vi "SGSA_Sweep_record_ALL.vi"() -> ()   [LabVIEW 2023, in "SG_SA.lvlib"]
uses:
  SG_SA.lvlib
  Clover_Cell.lvlib
panel:
  in  "Air_Loss":dbl=8.0
  in  "Cable_Loss":dbl=8.0
  in  "WaitingTime(ms)":u32=1000
  in  "FileNote":string
  in  "TRXmode":u16(ring)=1 items=["QUERY_TELEM_2 (V)"=2, "QUERY_TELEM_1 (H)"=1]
  out "SG Power (dBm)":i32
  in  "Stop Power":i32=8
  in  "Start Power":i32=-40
  in  "SG":refnum<visa-resource-name>="TCPIP0::192.168.100.200::inst0::INSTR"
  in  "SA":refnum<visa-resource-name>="TCPIP0::192.168.100.230::inst0::INSTR"
  in  "AvgTimes":i32=5
  out "Spectrum Data":dbl[](graph)
  out "AiP_8":dbl format="%#2.2f"
  out "AiP_7":dbl format="%#2.2f"
  out "AiP_6":dbl format="%#2.2f"
  out "AiP_5":dbl format="%#2.2f"
  out "AiP_4":dbl format="%#2.2f"
  out "AiP_3":dbl format="%#2.2f"
  out "AiP_2":dbl format="%#2.2f"
  out "AiP_1":dbl format="%#2.2f"
  # "Temperature"
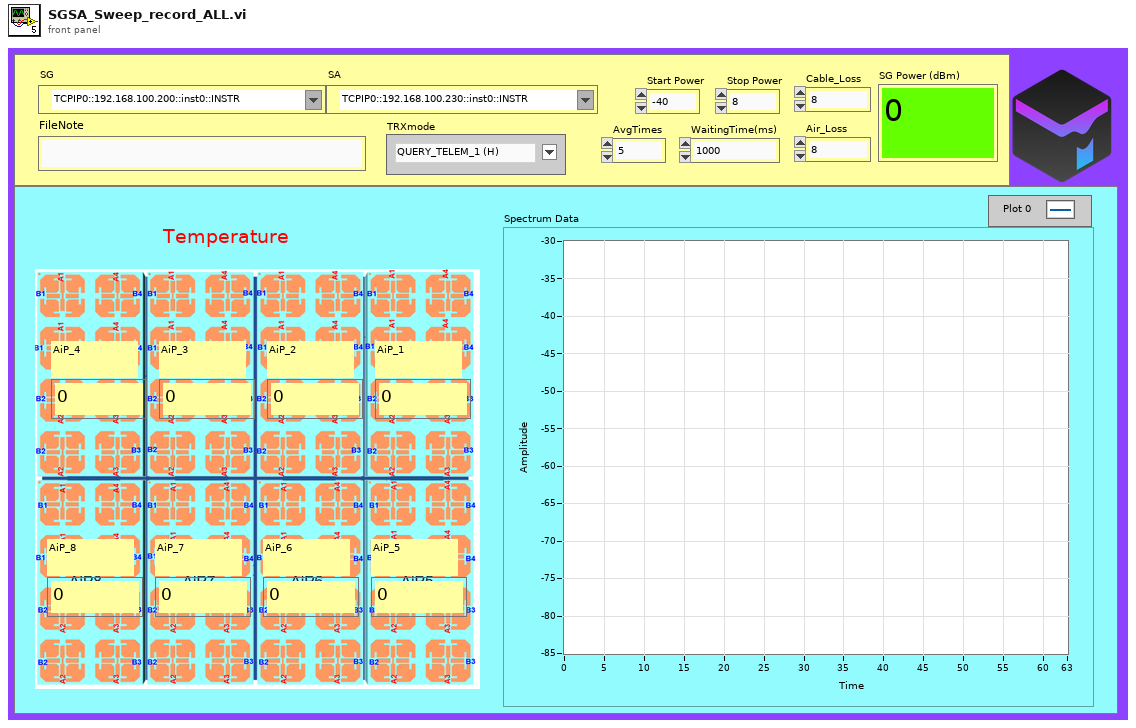
[diagram p1: front panel]
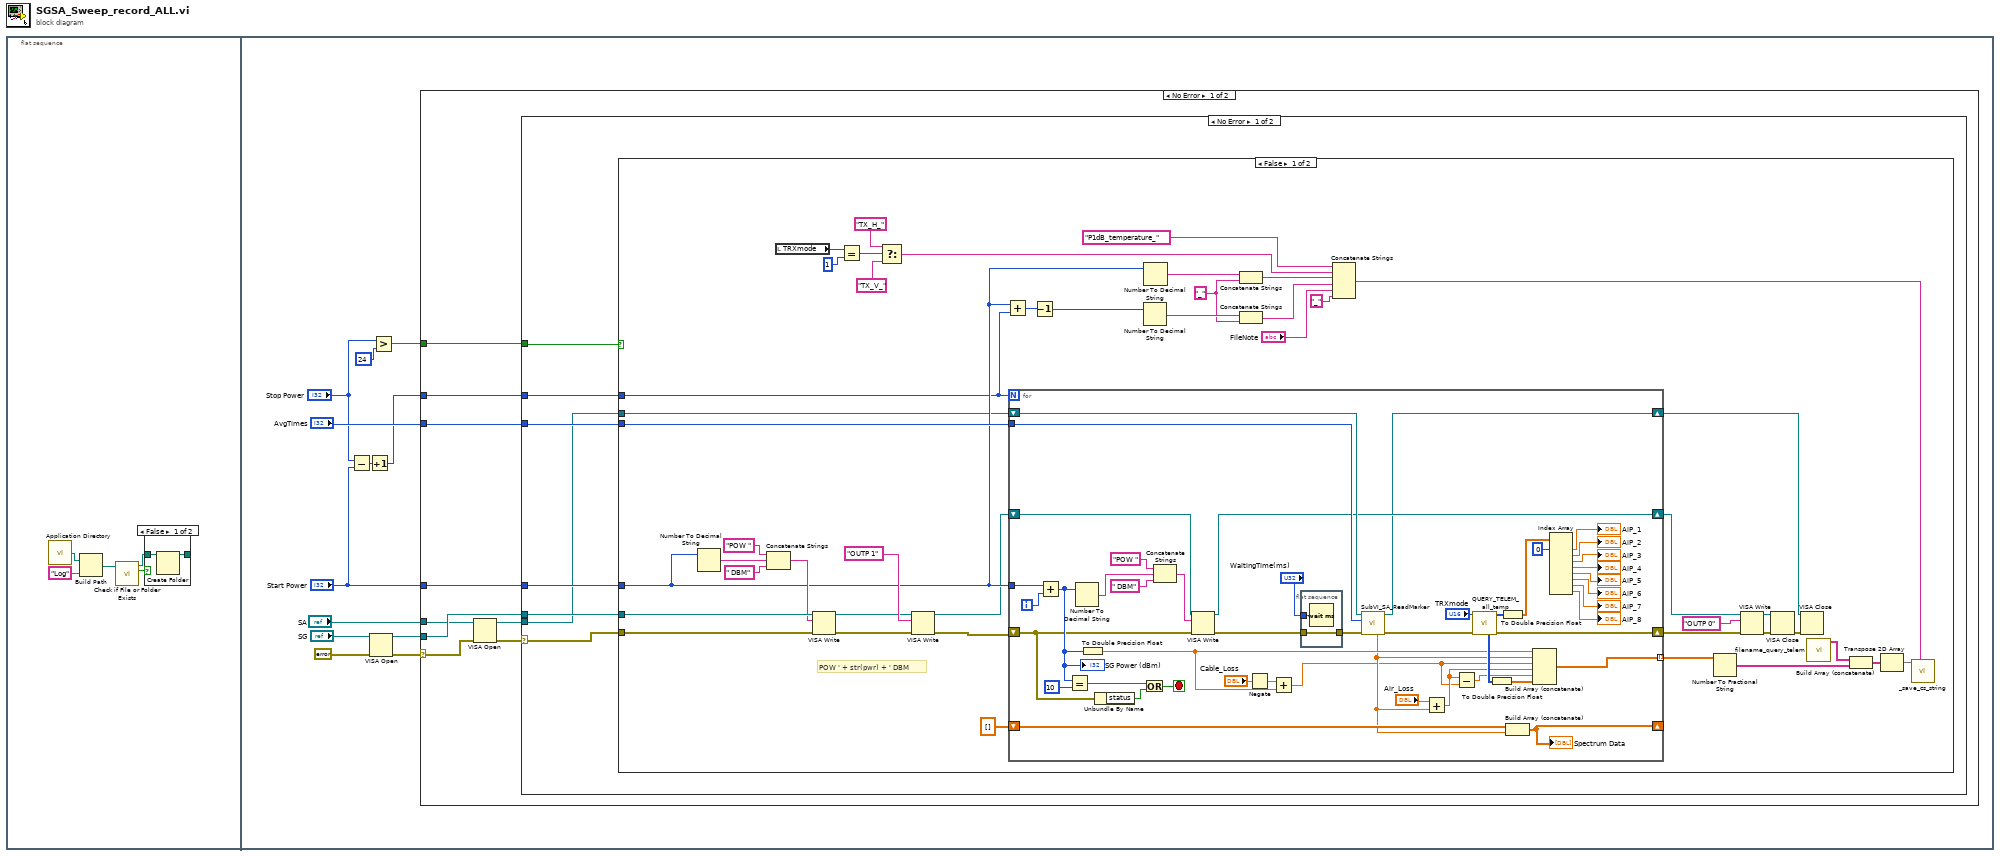
[diagram p0: block diagram]
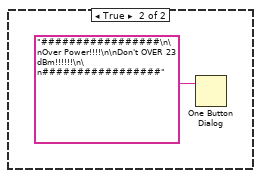
[diagram p3: hidden frame]
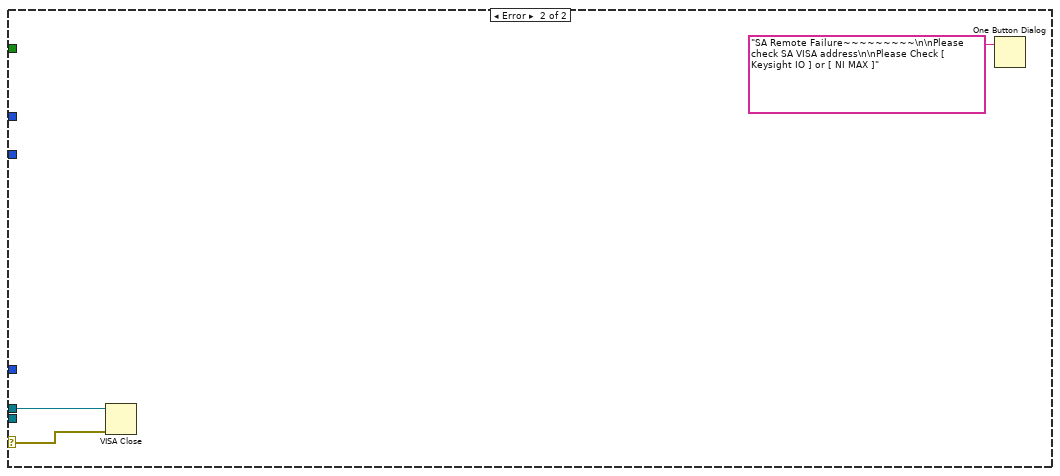
[diagram p4: hidden frame]
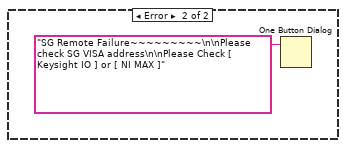
[diagram p5: hidden frame]
diagram:
  n1 = flat-sequence {
    frame #0 {
      n2 = call <vilib>:"Application Directory.vi"() -> ("Application Directory"=w4:path)
      n3 = Build Path(base path=w4, name or relative path="Log") -> (appended path=w1:path)
      n4 = call <vilib>:"Check if File or Folder Exists.vi"("path"=w1) -> ("file or folder exists?"=w3:bool, "dup path"=w2:path)  [unwired: 8 in, 1 out]
      n5 = case shown="False" w3 {
        tunnel: w2 -> [w7 w8]
        tunnel: [w6 w8] -> _
        frame False {
          n6 = Create Folder(path (use dialog)=w7) -> (created path=w6:path)  [unwired: 2 in, 2 out]
        }
        frame True {
        }
      }
    }
    frame #1 {
      n7 = Subtract(x="Stop Power", y="Start Power") -> (x-y=w17:i32)
      n8 = Increment(x=w17) -> (x+1=w16:i32)
      n9 = VISA Open(error in (no error)=errorcluster {"status"=FALSE, "code"=0, "source"=""}, VISA resource name="SG") -> (VISA resource name=w11:refnum<visa-resource-name>, error out=w9:errorcluster)  [unwired: 3 in]
      n10 = Greater?(x="Stop Power", y=24) -> (0:w20:bool)
      n11 = case shown="No Error" w9 {
        selector: w9 -> [w22 _]
        tunnel: w20 -> [w29 _]
        tunnel: "Start Power" -> [w28 _]
        tunnel: "AvgTimes" -> [w27 _]
        tunnel: w16 -> [w26 _]
        tunnel: w11 -> [w25 _]
        tunnel: "SA" -> [w24 _]
        frame No Error {
          n12 = VISA Open(error in (no error)=w22, VISA resource name=w24) -> (VISA resource name=w23:refnum<visa-resource-name>, error out=w21:errorcluster)  [unwired: 3 in]
          n13 = case shown="No Error" w21 {
            selector: w21 -> [w30 w132]
            tunnel: w29 -> [w36 _]
            tunnel: w28 -> [w35 _]
            tunnel: w27 -> [w34 _]
            tunnel: w26 -> [w33 _]
            tunnel: w25 -> [w32 w133]
            tunnel: w23 -> [w31 _]
            frame No Error {
              n14 = case shown="False" w36 {
                tunnel: w34 -> [w81 _]
                tunnel: w35 -> [w71 _]
                tunnel: w30 -> [w75 _]
                tunnel: w32 -> [w74 _]
                tunnel: w33 -> [w70 _]
                tunnel: w31 -> [w45 _]
                frame False {
                  w61 = "_"
                  # "POW ' + str(pwr) + ' DBM"
                  n15 = Number To Decimal String(number=w71) -> (decimal integer string=w77:string)  [unwired: 1 in]
                  n16 = Concatenate Strings("POW ", w77, " DBM") -> (w72:string)
                  n17 = local read "TRXmode"() -> (w44:u16)
                  n18 = VISA Write(VISA resource name=w74, write buffer=w72, error in (no error)=w75) -> (VISA resource name out=w73:refnum<visa-resource-name>, error out=w76:errorcluster)  [unwired: 1 out]
                  n19 = Equal?(x=w44, y=u16 1) -> (x = y?=w42:bool)
                  n20 = Select(t="TX_H_" ("delimiter (\\t)"), s=w42, f="TX_V_" ("delimiter (\\t)")) -> (s? t:f=w39:string)
                  n21 = VISA Write(VISA resource name=w73, write buffer="OUTP 1", error in (no error)=w76) -> (VISA resource name out=w69:refnum<visa-resource-name>, error out=w68:errorcluster)  [unwired: 1 out]
                  n22 = Add(x=w71, y=w70) -> (x+y=w65:i32)
                  n23 = for {
                    N: w70 -> [_]
                    tunnel: w81 -> [w127]
                    tunnel: w71 -> [w125]
                    tunnel: [w120] -> w53 mode=indexing
                    shift-right: [w116] -> w66
                    shift-left: w68 -> [w100]
                    shift-right: [w113] -> w58
                    shift-left: w69 -> [w112]
                    shift-right: [w96] -> w46
                    shift-left: w45 -> [w128]
                    shift-right: [w91] -> _
                    shift-left: dbl[] [] -> [w92]
                    i -> [w126]
                    stop <- w99 stop-if-true
                    n24 = Add(x=w125, y=w126) -> (x+y=w119:i32)
                    "SG Power (dBm)" <- w119
                    n25 = Equal?(x=w119, y=10) -> (x = y?=w98:bool)
                    n26 = Number To Decimal String(number=w119) -> (decimal integer string=w122:string)  [unwired: 1 in]
                    n27 = To Double Precision Float(number=w119) -> (double precision float=w88:dbl)
                    n28 = Unbundle By Name(w100) -> ("status"=w97:bool)
                    n29 = Or(x=w98, y=w97) -> (x .or. y?=w99:bool)
                    n30 = Concatenate Strings("POW ", w122, " DBM") -> (w121:string)
                    n31 = VISA Write(VISA resource name=w112, write buffer=w121, error in (no error)=w100) -> (VISA resource name out=w113:refnum<visa-resource-name>, error out=w95:errorcluster)  [unwired: 1 out]
                    n32 = Negate(x="Cable_Loss") -> (-x=w89:dbl)
                    n33 = Add(x=w89, y=w88) -> (x+y=w83:dbl)
                    n34 = flat-sequence {
                      tunnel: w95 -> [w130]
                      tunnel: [w130] -> w94
                      tunnel: "WaitingTime(ms)" -> [w129]
                      frame #0 {
                        n35 = Wait (ms)(milliseconds to wait=w129) -> ()  [unwired: 1 out]
                      }
                    }
                    n36 = call "SubVI_SA_ReadMarker.vi"("error in (no error)"=w94, "AvgTimes"=w127, "VISA resource name"=w128) -> ("error out"=w117:errorcluster, "VISA resource name out"=w96:refnum<visa-resource-name>, "Marker Power"=w86:dbl)  [unwired: 5 in, 1 out]
                    n37 = Add(x="Air_Loss", y=w86) -> (x+y=w84:dbl)
                    n38 = Subtract(x=w84, y=w83) -> (x-y=w82:dbl)
                    n39 = call "QUERY_TELEM_all_temp.vi"("error in"=w117, "TRXmode"="TRXmode") -> ("error out"=w116:errorcluster, "Temp_8pcs"=w115:i32[], "all_data"=w101:i32[])  [unwired: 7 in]
                    n40 = To Double Precision Float(number=w101) -> (double precision float=w85:dbl[])
                    n41 = To Double Precision Float(number=w115) -> (double precision float=w111:dbl[])
                    n42 = Build Array (concatenate)(w92, w86) -> (w91:dbl[])
                    "Spectrum Data" <- w91
                    n43 = Build Array (concatenate)(w88, w86, w83, w84, w82, w85) -> (w120:dbl[])
                    n44 = Index Array(array=w111, index #1=0 ("index")) -> (element #1=→"AiP_1":dbl, element #2=→"AiP_2":dbl, element #3=→"AiP_3":dbl, element #4=→"AiP_4":dbl, element #5=→"AiP_5":dbl, element #6=→"AiP_6":dbl, element #7=→"AiP_7":dbl, element #8=→"AiP_8":dbl)  [unwired: 7 in]
                  }
                  n45 = Decrement(x=w65) -> (x-1=w64:i32)
                  n46 = Number To Decimal String(number=w64) -> (decimal integer string=w62:string)  [unwired: 1 in]
                  n47 = Number To Decimal String(number=w71) -> (decimal integer string=w63:string)  [unwired: 1 in]
                  n48 = Concatenate Strings(w63, w61) -> (w60:string)
                  n49 = Concatenate Strings(w62, w61) -> (w59:string)
                  n50 = Concatenate Strings("P1dB_temperature_" ("delimiter (\\t)"), w39, w60, w59, "FileNote", "_") -> (w52:string)
                  n51 = Number To Fractional String(number=w53) -> (F-format string=w54:string[][])  [unwired: 3 in]
                  n52 = VISA Write(VISA resource name=w58, write buffer="OUTP 0", error in (no error)=w66) -> (VISA resource name out=w48:refnum<visa-resource-name>, error out=w49:errorcluster)  [unwired: 1 out]
                  n53 = VISA Close(VISA resource name=w48, error in (no error)=w49) -> (error out=w47:errorcluster)
                  n54 = VISA Close(VISA resource name=w46, error in (no error)=w47) -> ()  [unwired: 1 out]
                  n55 = call "filename_query_telem.vi"() -> ("appended array"=w50:string[][])  [unwired: 11 in]
                  n56 = Build Array (concatenate)(w50, w54) -> (w55:string[][])
                  n57 = Transpose 2D Array(2D array=w55) -> (transposed array=w51:string[][])
                  n58 = call "_save_cs_string.vi"("FileName"=w52, "Array"=w51) -> ()  [unwired: 9 in, 1 out]
                }
                frame True {
                  n59 = One Button Dialog(message="#################\n\nOver Power!!!!\n\nDon't OVER 23 dBm!!!!!!\n\n#################") -> ()  [unwired: 1 in, 1 out]
                }
              }
            }
            frame Error {
              n60 = VISA Close(VISA resource name=w133, error in (no error)=w132) -> ()  [unwired: 1 out]
              n61 = One Button Dialog(message="SA Remote Failure~~~~~~~~~\n\nPlease check SA VISA address\n\nPlease Check [ Keysight IO ] or [ NI MAX ]") -> ()  [unwired: 1 in, 1 out]
            }
          }
        }
        frame Error {
          n62 = One Button Dialog(message="SG Remote Failure~~~~~~~~~\n\nPlease check SG VISA address\n\nPlease Check [ Keysight IO ] or [ NI MAX ]") -> ()  [unwired: 1 in, 1 out]
        }
      }
    }
  }
